vi "When Dummy.vi"(0 "error out":errorcluster, 2 "Boolean":bool, 11 "Test Interface in":refnum<class "Test Interface Mock.lvclass">) -> (3 "Test Interface out":refnum<class "Test Interface Mock.lvclass">)   [LabVIEW 2020, in "Test Interface Mock.lvclass"]
uses:
  Test Interface Mock.lvclass
  Test Interface Mock.lvclass/Test Interface Mock.ctl
  <vilib>/Astemes/LMock/Mock.lvclass
  C:/Program Files (x86)/National Instruments/LabVIEW 2020/vi.lib/Astemes/LMock/Mock.lvclass
  C:/git/astemes-lmock/sandbox/Benchmark/Test Interface Mock/Test Interface Mock.lvclass
  C:/git/astemes-lmock/sandbox/Benchmark/Test Interface/Test Interface.lvclass
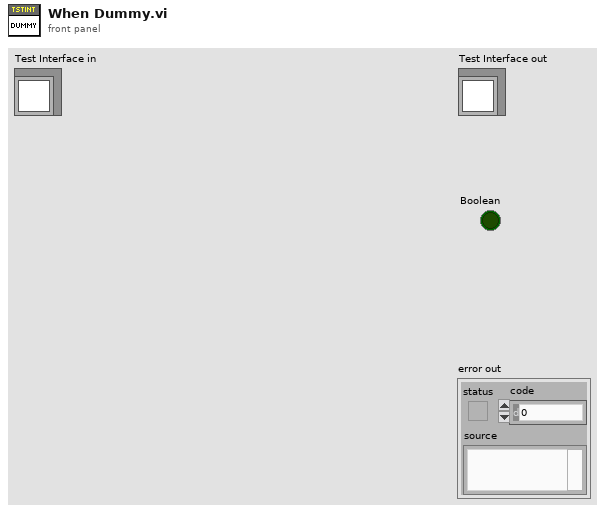
[diagram p1: front panel]
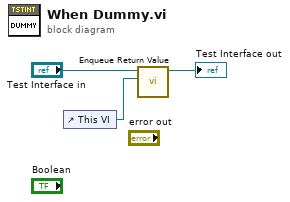
[diagram p0: block diagram]
diagram:
  n1 = control-ref of="This VI"() -> (w1:refnum<vi>)
  n2 = call <vilib>:"Enqueue Return Value.vi"("This VI"=w1, "Mock In"="Test Interface in") -> ("Mock Out"=→"Test Interface out":refnum<class "Test Interface Mock.lvclass">)  [unwired: 8 in, 1 out]
